vi "Get Image Data.vi"(8 "error in (no error)":errorcluster, 11 "ImageData":refnum<k24>) -> (0 "error out":errorcluster, 1 "ImageDataFormat":i32(ring) items=["BGRPlanar", "BGRPixel", "RGBPixel", "Monochrome"], 2 "BitDepth":i32, 3 "Frame Data":u16[][][](array[numeric]))   [LabVIEW 2015]
uses:
  C:/code/Host/Installer/Scientific Camera Interfaces/LabVIEW/64_bit/Library_X64/Thorlabs.TSI.ImageDataInterfaces.dll
  64_bit/Library_X64/Thorlabs.TSI.ImageDataInterfaces.dll
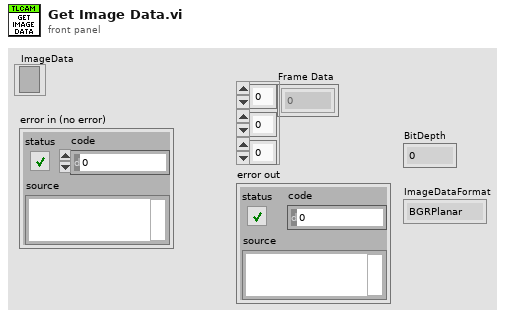
[diagram p1: front panel]
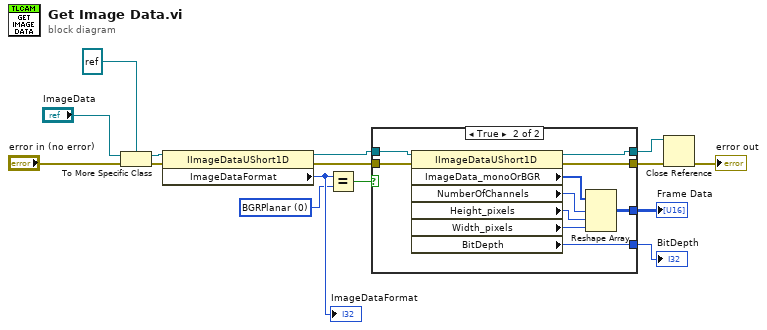
[diagram p0: block diagram]
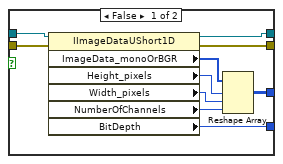
[diagram p2: hidden frame]
diagram:
  w5 = 0 items=["BGRPlanar", "BGRPixel", "RGBPixel", "Monochrome"] ("ImageDataFormat")
  n1 = To More Specific Class(target class=refnum<k24> refnum, reference="ImageData", error in="error in (no error)") -> (specific class reference=w10:refnum<k24>, error out=w9:errorcluster)
  n2 = property class="IImageDataUShort1D"(reference=w10, error in=w9) -> (reference out=w8:refnum<k24>, error out=w7:errorcluster, "ImageDataFormat"=w6:i32)
  "ImageDataFormat" <- w6
  n3 = Equal?(x=w6, y=w5) -> (x = y?=w4:bool)
  n4 = case shown="True" w4 {
    tunnel: [w25 w35] -> w15
    tunnel: [w24 w34] -> w14
    tunnel: [w23 w33] -> w12
    tunnel: [w22 w32] -> w11
    tunnel: w8 -> [w21 w31]
    tunnel: w7 -> [w20 w30]
    frame False {
      n5 = property class="IImageDataUShort1D"(reference=w21, error in=w20) -> (reference out=w24:refnum<k24>, error out=w25:errorcluster, "ImageData_monoOrBGR"=w19:u16[], "Height_pixels"=w17:i32, "Width_pixels"=w18:i32, "NumberOfChannels"=w16:i32, "BitDepth"=w22:i32)
      n6 = Reshape Array(w19, w17, w18, w16) -> (w23:u16[][][])
    }
    frame True {
      n7 = property class="IImageDataUShort1D"(reference=w31, error in=w30) -> (reference out=w34:refnum<k24>, error out=w35:errorcluster, "ImageData_monoOrBGR"=w29:u16[], "NumberOfChannels"=w27:i32, "Height_pixels"=w28:i32, "Width_pixels"=w26:i32, "BitDepth"=w32:i32)
      n8 = Reshape Array(w29, w27, w28, w26) -> (w33:u16[][][])
    }
  }
  "Frame Data" <- w12
  "BitDepth" <- w11
  n9 = Close Reference(reference=w14, error in (no error)=w15) -> (error out=→"error out":errorcluster)
